vi "FTW-Test-JSON-ObjectKeys.vi"() -> (0 "Test Result":errorcluster)   [LabVIEW 2014]
uses:
  src/core/error/FTW-ERR-Assert-DeveloperError.vi
  src/core/error/FTW-ERR-ThrowError.vi
  src/core/error/FTW-ERR-CallChain.vi
  src/core/string/FTW-STR-ReplaceWhitespace.vi
panel:
  out "JSON String (UTF-8)":string
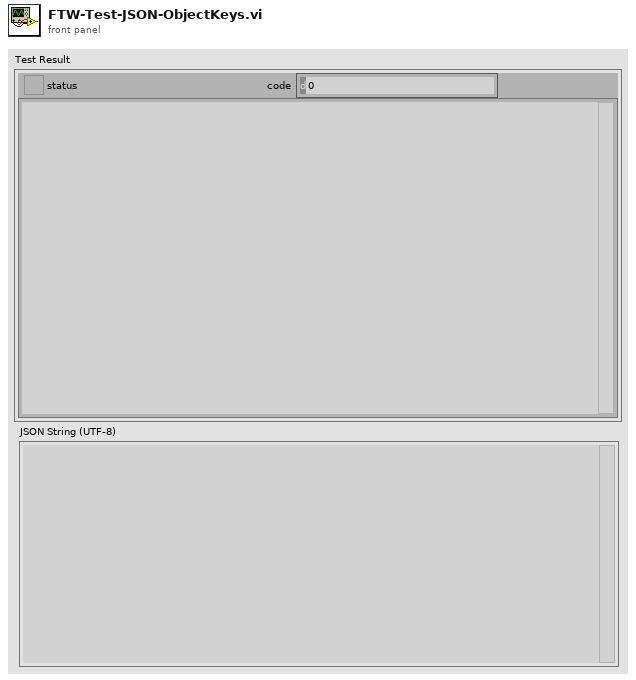
[diagram p1: front panel]
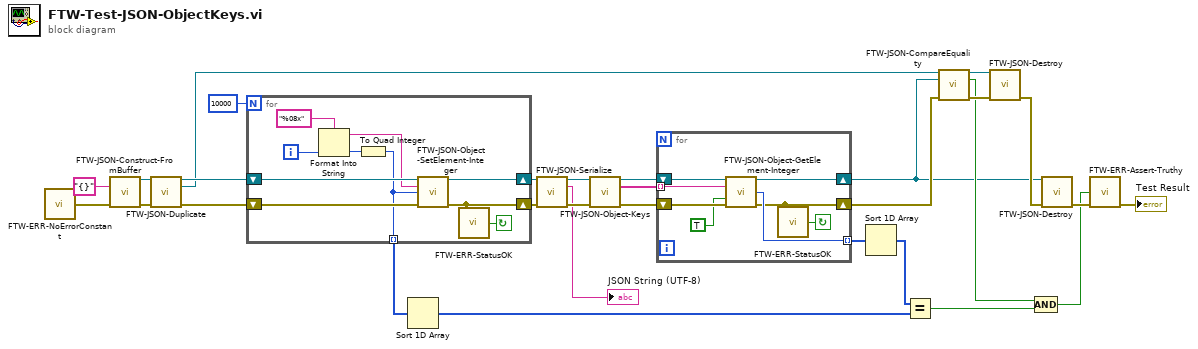
[diagram p0: block diagram]
diagram:
  n1 = call "FTW-ERR-NoErrorConstant.vi"() -> ("no error"=w29:errorcluster)
  n2 = call "FTW-JSON-Construct-FromBuffer.vi"("JSON String (UTF-8)"="{}", "error in"=w29) -> ("JSON Object"=w25:refnum<data-value>, "error out"=w23:errorcluster)  [unwired: 12 in]
  n3 = call "FTW-JSON-Duplicate.vi"("JSON Object"=w25, "error in"=w23) -> ("JSON Object out"=w24:refnum<data-value>, "Duplicated JSON Object"=w18:refnum<data-value>, "error out"=w22:errorcluster)  [unwired: 11 in]
  n4 = for {
    N: 10000 -> [_]
    shift-right: [w32] -> w9
    shift-left: w22 -> [w37]
    shift-right: [w38] -> w11
    shift-left: w24 -> [w39]
    tunnel: [w33] -> w4 mode=indexing
    i -> [w36]
    stop <- w31 continue-if-true
    n5 = Format Into String(format string="%08x", w36) -> (resulting string=w35:string)  [unwired: 2 in, 1 out]
    n6 = To Quad Integer(1:w36) -> (0:w33:i64)
    n7 = call "FTW-JSON-Object-SetElement-Integer.vi"("JSON Object"=w39, "Key"=w35, "Value"=w33, "error in"=w37) -> ("JSON Object out"=w38:refnum<data-value>, "error out"=w32:errorcluster)  [unwired: 10 in]
    n8 = call "FTW-ERR-StatusOK.vi"("error to check"=w32) -> ("Status OK?"=w31:bool)
  }
  n9 = Sort 1D Array(array=w4) -> (sorted array=w3:i64[])
  n10 = call "FTW-JSON-Serialize.vi"("JSON Object"=w11, "error in"=w9) -> ("JSON Object out"=w10:refnum<data-value>, "JSON String (UTF-8)"=→"JSON String (UTF-8)":string, "error out"=w8:errorcluster)  [unwired: 11 in]
  n11 = call "FTW-JSON-Object-Keys.vi"("JSON Object"=w10, "error in"=w8) -> ("JSON Object out"=w28:refnum<data-value>, "Keys"=w27:string[], "error out"=w26:errorcluster)  [unwired: 11 in]
  n12 = for {
    tunnel: w27 -> [w45] mode=indexing
    shift-right: [w41] -> w16
    shift-left: w26 -> [w46]
    tunnel: [w44] -> w6 mode=indexing
    shift-right: [w43] -> w1
    shift-left: w28 -> [w47]
    stop <- w42 continue-if-true
    n13 = call "FTW-JSON-Object-GetElement-Integer.vi"("JSON Object"=w47, "Key"=w45, "Consume Value"=TRUE, "error in"=w46) -> ("JSON Object out"=w43:refnum<data-value>, "Value"=w44:i64, "error out"=w41:errorcluster)  [unwired: 8 in, 1 out]
    n14 = call "FTW-ERR-StatusOK.vi"("error to check"=w41) -> ("Status OK?"=w42:bool)
  }
  n15 = Sort 1D Array(array=w6) -> (sorted array=w5:i64[])
  n16 = Equal?(x=w5, y=w3) -> (x = y?=w13:bool)
  n17 = call "FTW-JSON-CompareEquality.vi"("JSON Object"=w18, "JSON Object to Compare"=w1, "error in"=w16) -> ("JSON Object out"=w2:refnum<data-value>, "Equal?"=w14:bool, "error out"=w17:errorcluster)  [unwired: 10 in]
  n18 = call "FTW-JSON-Destroy.vi"("JSON Object"=w2, "error in"=w17) -> ("error out"=w15:errorcluster)  [unwired: 13 in]
  n19 = Compound Arithmetic op=AND(w14, w13) -> (w12:bool)
  n20 = call "FTW-JSON-Destroy.vi"("JSON Object"=w1, "error in"=w15) -> ("error out"=w20:errorcluster)  [unwired: 13 in]
  n21 = call "FTW-ERR-Assert-Truthy.vi"("Expected Truthy"=w12, "error in"=w20) -> ("error out"=→"Test Result":errorcluster)  [unwired: 13 in]
